vi "RSZVB Set Physical Port Resolution Bandwidth.vi"(7 "Resolution Bandwidth (10.0E+3)":dbl=10000.0 format="%^.3e", 8 "error in (no error)":errorcluster {"code" format="%.0x"}, 9 "Analyzer Port (1)":i32=1, 10 "Channel (1)":i32=1, 11 "VISA session":refnum<visa-resource-name>) -> (0 "error out":errorcluster {"code" format="%.0x"}, 3 "dup VISA session":refnum<visa-resource-name>)   [LabVIEW 2011]
doc: "Defines the resolution bandwidth of the analyzer for all partial measurements where an analyzer source port <Pt> is used.\n\nRemote-control command(s):\n[SENSe<Ch>:]BANDwidth|BWIDth[:RESolution]:PORT<Pt>"
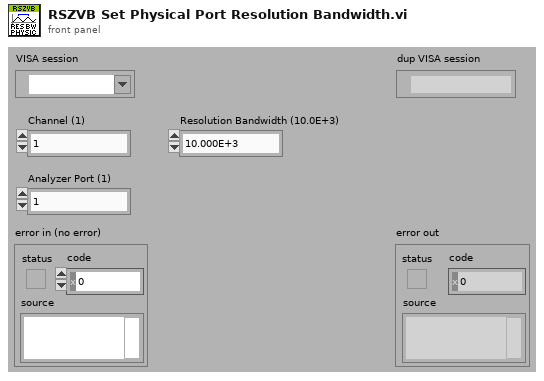
[diagram p1: front panel]
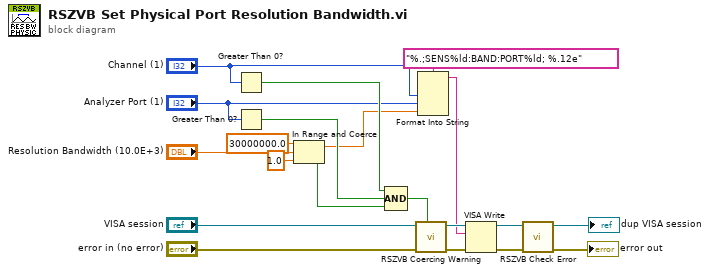
[diagram p0: block diagram]
diagram:
  n1 = Greater Than 0?(x="Channel (1)") -> (x > 0?=w14:bool)
  n2 = Greater Than 0?(x="Analyzer Port (1)") -> (x > 0?=w13:bool)
  n3 = In Range and Coerce(upper limit=30000000.0, x="Resolution Bandwidth (10.0E+3)", lower limit=1.0) -> (coerced(x)=w10:dbl, In Range?=w11:bool)
  n4 = Compound Arithmetic op=AND(w14, w13, w11) -> (w12:bool)
  n5 = call "RSZVB Coercing Warning.vi"("In Range?"=w12, "error in (no error)"="error in (no error)", "VISA session"="VISA session") -> ("error out"=w18:errorcluster, "dup VISA session"=w19:refnum<visa-resource-name>)  [unwired: 7 in]
  n6 = Format Into String(format string="%.;SENS%ld:BAND:PORT%ld; %.12e", "Channel (1)", "Analyzer Port (1)", w10) -> (resulting string=w15:string)  [unwired: 2 in, 1 out]
  n7 = VISA Write(VISA resource name=w19, write buffer=w15, error in (no error)=w18) -> (VISA resource name out=w16:refnum<visa-resource-name>, error out=w17:errorcluster)  [unwired: 1 out]
  n8 = call "RSZVB Check Error.vi"("error in (no error)"=w17, "VISA session"=w16) -> ("error out"=→"error out":errorcluster, "dup VISA session"=→"dup VISA session":refnum<visa-resource-name>)  [unwired: 8 in]
